vi "optionsAcq_spectrumType.vi"(8 "error in (no error)":errorcluster, 9 "readWrite":enum16{"read", "write"}(ring), 10 "spectrum channel type":T1, 11 "Thorlabs_OSA_64 in":refnum<class "OSA.lvclass">) -> (0 "error out":errorcluster, 2 "spectrum channel out":T1, 3 "Thorlabs_OSA_64 out":refnum<class "OSA.lvclass">)   [LabVIEW 2010, in "OSA.lvclass"]
uses:
  OSA.lvclass
  _misc/Thorlabs_FTS_misc.llb/channelType_spectrum.ctl
  OSA20X_misc.lvlib
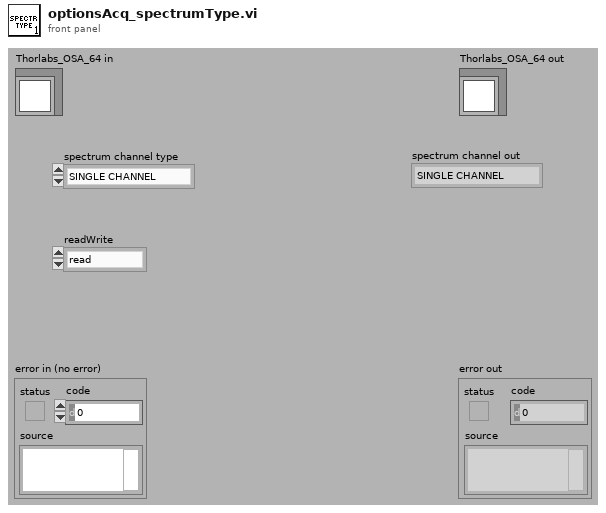
[diagram p1: front panel]
types:
  T1 = typedef "OSA20X_misc.lvlib/channelType_spectrum.ctl" = enum16{"SINGLE CHANNEL", "STICHED"}
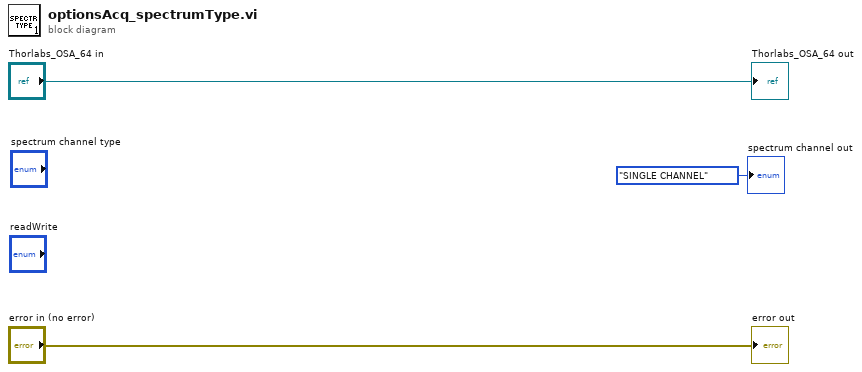
[diagram p0: block diagram]
diagram:
  "error out" <- "error in (no error)"
  "Thorlabs_OSA_64 out" <- "Thorlabs_OSA_64 in"
  "spectrum channel out" <- channelType_spectrum."SINGLE CHANNEL" ("spectrum channel out")
